vi "MaxiumCentered.vi"(9 "Buffer":dbl, 10 "Number of Points":dbl, 11 "Input Y Values":dbl[](array[numeric])) -> (2 "State output":T1(ring), 3 "Output Y Values":dbl[](array[numeric]))   [LabVIEW 2014]
panel:
  # "CenterMax VI"
  # "Is the Waveform Peak in the Middle?"
  # "Inputs"
  # "Outputs"
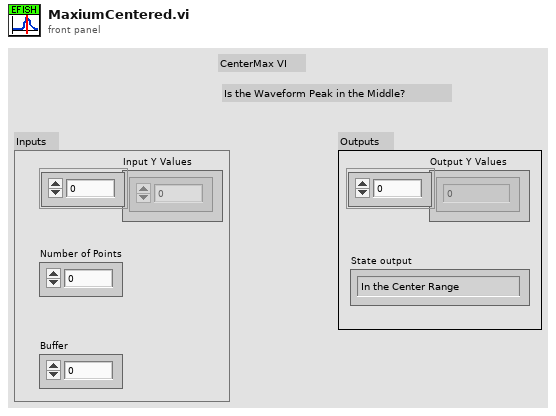
[diagram p1: front panel]
types:
  T1 = enum16{"In the Center Range", "Before the Center Range", "After the Center Range"}
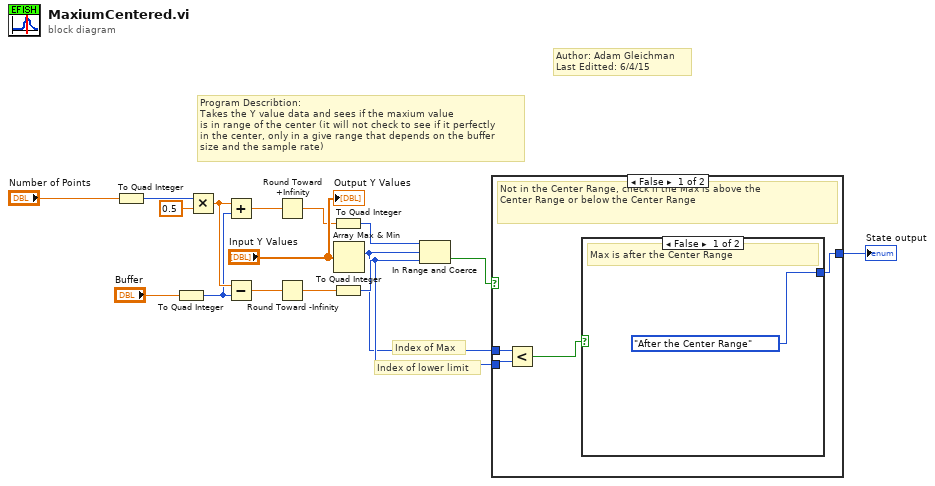
[diagram p0: block diagram]
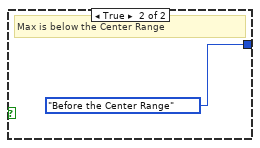
[diagram p2: hidden frame]
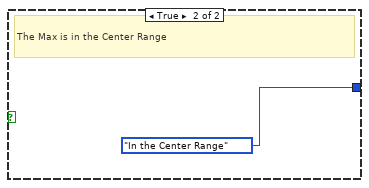
[diagram p3: hidden frame]
diagram:
  # "Index of lower limit"
  # "Index of Max"
  # "Program Describtion: \nTakes the Y value data and sees if the maxium value\nis in range of the center (it will not check to see if it perfectly\nin the center, only in a give range that depends on the buffer\nsize and the sample rate)"
  # "Author: Adam Gleichman\nLast Editted: 6/4/15"
  n1 = To Quad Integer(1:"Number of Points") -> (0:w13:i64)
  n2 = To Quad Integer(1:"Buffer") -> (0:w8:i64)
  n3 = Multiply(x=w13, y=0.5) -> (x*y=w9:dbl)
  n4 = Add(x=w9, y=w8) -> (x+y=w7:dbl)
  n5 = Subtract(x=w9, y=w8) -> (x-y=w11:dbl)
  n6 = Round Toward +Infinity(x=w7) -> (ceil(x): smallest int >= x=w6:dbl)
  n7 = Round Toward -Infinity(1:w11) -> (0:w10:dbl)
  n8 = To Quad Integer(1:w6) -> (0:w5:i64)
  n9 = To Quad Integer(1:w10) -> (0:w2:i64)
  n10 = Array Max & Min(array="Input Y Values") -> (max index (indices)=w1:i32)  [unwired: 3 out]
  n11 = In Range and Coerce(upper limit=w5, x=w1, lower limit=w2) -> (In Range?=w4:bool)  [unwired: 1 out]
  n12 = case shown="False" w4 {
    tunnel: [w17 T1."In the Center Range" ("something")] -> w3
    tunnel: w2 -> [w19 _]
    tunnel: w1 -> [w20 _]
    frame False {
      # "Not in the Center Range, check if the Max is above the \nCenter Range or below the Center Range"
      n13 = Less?(x=w20, y=w19) -> (x < y?=w18:bool)
      n14 = case shown="False" w18 {
        tunnel: [T1."After the Center Range" ("something") T1."Before the Center Range" ("something")] -> w17
        frame False {
          # "Max is after the Center Range"
        }
        frame True {
          # "Max is below the Center Range"
        }
      }
    }
    frame True {
      # "The Max is in the Center Range"
    }
  }
  "State output" <- w3
  "Output Y Values" <- "Input Y Values"
